vi "Detector Setup.vi"(8 "error in (no error)":errorcluster, 11 "RIMAS Detector in":refnum<class "RIMAS Detector.lvclass">) -> (0 "error out":errorcluster, 2 "Detector Config.Detector":u16, 3 "RIMAS Detector out":refnum<class "RIMAS Detector.lvclass">)   [LabVIEW 2024, in "RIMAS Detector.lvclass"]
uses:
  RIMAS Detector.lvclass
  RIMAS Detector.lvclass/RIMAS Detector.ctl
  Detector Class.lvclass
panel:
  out "data out 2":string
  out "data out":string
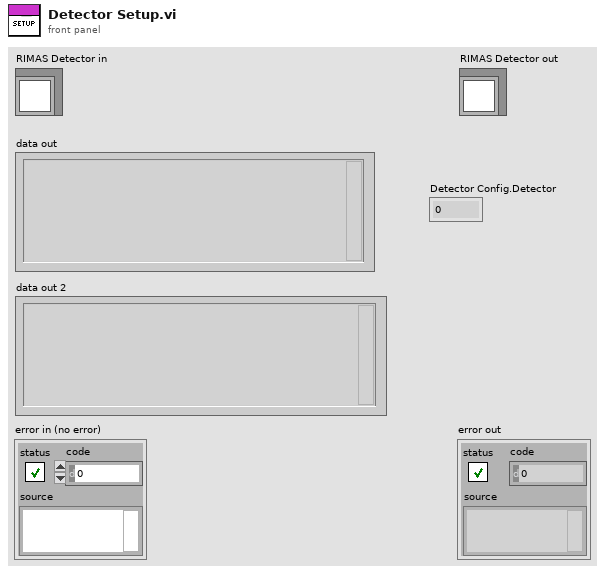
[diagram p1: front panel]
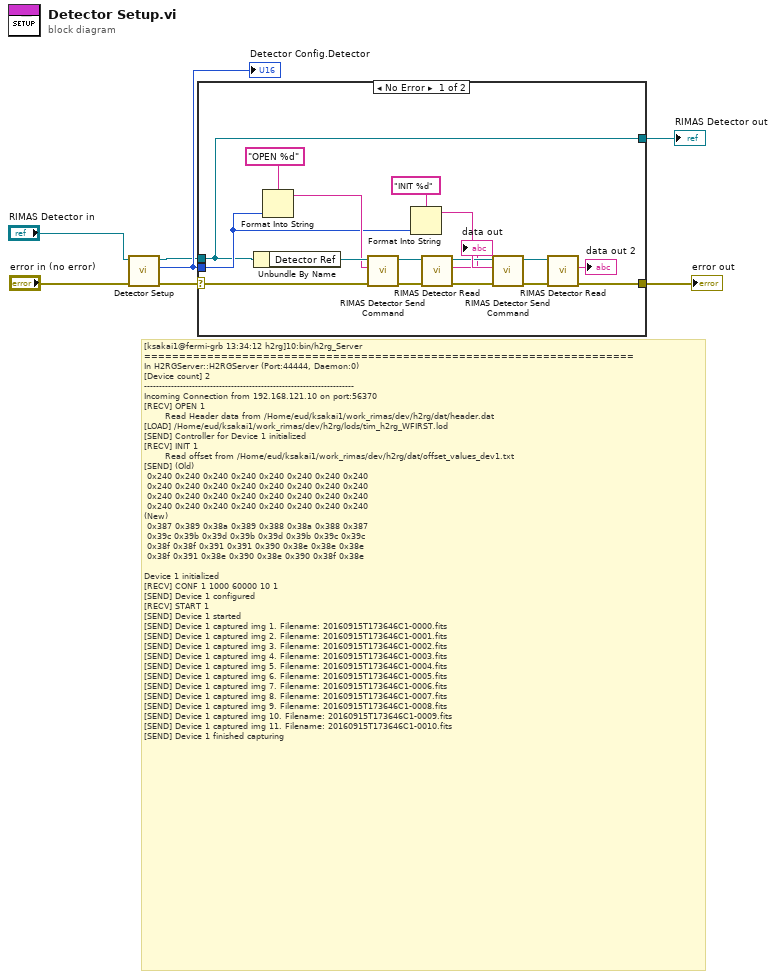
[diagram p0: block diagram]
diagram:
  # "[ksakai1@fermi-grb 13:34:12 h2rg]10:bin/h2rg_Server\n======================================================================\nIn H2RGServer::H2RGServer (Port:44444, Daemon:0)\n[Device count] 2\n----------------------------------------------------------------------\nIncoming Connection from 192.168.121.10 on port:56370\n[RECV] OPEN 1\n       Read Header data from /Home/eud/ksakai1/work_rimas/dev/h2rg/dat/header.dat\n[LOAD] /Home/eud/ksakai1/work_rimas/dev/h2rg/lods/tim_h2rg_WFIRST.lod\n[SEND] Controller for Device 1 initialized\n[RECV] INIT 1\n       Read offset from /Home/eud/ksakai1/work_rimas/dev/h2rg/dat/offset_values_dev1.txt\n[SEND] (Old)\n 0x240 0x240 0x240 0x240 0x240 0x240 0x240 0x240\n 0x240 0x240 0x240 0x240 0x240 0x240 0x240 0x240\n 0x240 0x240 0x240 0x240 0x240 0x240 0x240 0x240\n 0x240 0x240 0x240 0x240 0x240 0x240 0x240 0x240\n(New)\n 0x387 0x389 0x38a 0x389 0x388 0x38a 0x388 0x387\n 0x39c 0x39b 0x39d 0x39b 0x39d 0x39b 0x39c 0x39c\n 0x38f 0x38f 0x391 0x391 0x390 0x38e 0x38e 0x38e\n 0x38f 0x391 0x38e 0x390 0x38e 0x390 0x38f 0x38e\n\nDevice 1 initialized\n[RECV] CONF 1 1000 60000 10 1\n[SEND] Device 1 configured\n[RECV] START 1\n[SEND] Device 1 started\n[SEND] Device 1 captured img 1. Filename: 20160915T173646C1-0000.fits\n[SEND] Device 1 captured img 2. Filename: 20160915T173646C1-0001.fits\n[SEND] Device 1 captured img 3. Filename: 20160915T173646C1-0002.fits\n[SEND] Device 1 captured img 4. Filename: 20160915T173646C1-0003.fits\n[SEND] Device 1 captured img 5. Filename: 20160915T173646C1-0004.fits\n[SEND] Device 1 captured img 6. Filename: 20160915T173646C1-0005.fits\n[SEND] Device 1 captured img 7. Filename: 20160915T173646C1-0006.fits\n[SEND] Device 1 captured img 8. Filename: 20160915T173646C1-0007.fits\n[SEND] Device 1 captured img 9. Filename: 20160915T173646C1-0008.fits\n[SEND] Device 1 captured img 10. Filename: 20160915T173646C1-0009.fits\n[SEND] Device 1 captured img 11. Filename: 20160915T173646C1-0010.fits\n[SEND] Device 1 finished capturing"
  n1 = call-parent "Detector Setup.vi"("error in (no error)"="error in (no error)", "Detector Class in"="RIMAS Detector in") -> ("error out"=w5:errorcluster, "Detector Config.Detector"=w4:u16, "Detector Class out"=w3:refnum<class "RIMAS Detector.lvclass">)  [unwired: 7 in]
  "Detector Config.Detector" <- w4
  n2 = case shown="No Error" w5 {
    selector: w5 -> [w22 w25]
    tunnel: w4 -> [w20 _]
    tunnel: w3 -> [w17 w26]
    tunnel: [w8 w25] -> w2
    tunnel: [w17 w26] -> w1
    frame No Error {
      n3 = Unbundle By Name(w17) -> ("Detector Ref"=w23:refnum<k5>)
      n4 = Format Into String(format string="OPEN %d", w20) -> (resulting string=w21:string)  [unwired: 2 in, 1 out]
      n5 = call "RIMAS Detector Send Command.vi"("Error In"=w22, "Command"=w21, "Detector Ref"=w23) -> ("Error Out"=w15:errorcluster, "Detector Ref dup"=w16:refnum<k5>)  [unwired: 6 in, 1 out]
      n6 = Format Into String(format string="INIT %d", w20) -> (resulting string=w19:string)  [unwired: 2 in, 1 out]
      n7 = call "RIMAS Detector Read.vi"("Error In"=w15, "Detector Ref"=w16) -> ("Error Out"=w13:errorcluster, "data out"=→"data out":string, "Detector Ref dup"=w14:refnum<k5>)  [unwired: 6 in, 1 out]
      n8 = call "RIMAS Detector Send Command.vi"("Error In"=w13, "Command"=w19, "Detector Ref"=w14) -> ("Error Out"=w12:errorcluster, "Detector Ref dup"=w11:refnum<k5>)  [unwired: 6 in, 1 out]
      n9 = call "RIMAS Detector Read.vi"("Error In"=w12, "Detector Ref"=w11) -> ("Error Out"=w8:errorcluster, "data out"=→"data out 2":string)  [unwired: 6 in, 2 out]
    }
    frame Error {
    }
  }
  "error out" <- w2
  "RIMAS Detector out" <- w1
